vi "Protocol properties.vi"(11 "error in (no error)":errorcluster) -> (8 "LEIN system infor":T1={"STAT system size"=[6, 4, 2, 0, 0, 0, 0, 0, 0, 0, 0, 0, 0, 0, 18, 10]}, 15 "error out":errorcluster)   [LabVIEW 2010]
uses:
  Protocol properties.ctl
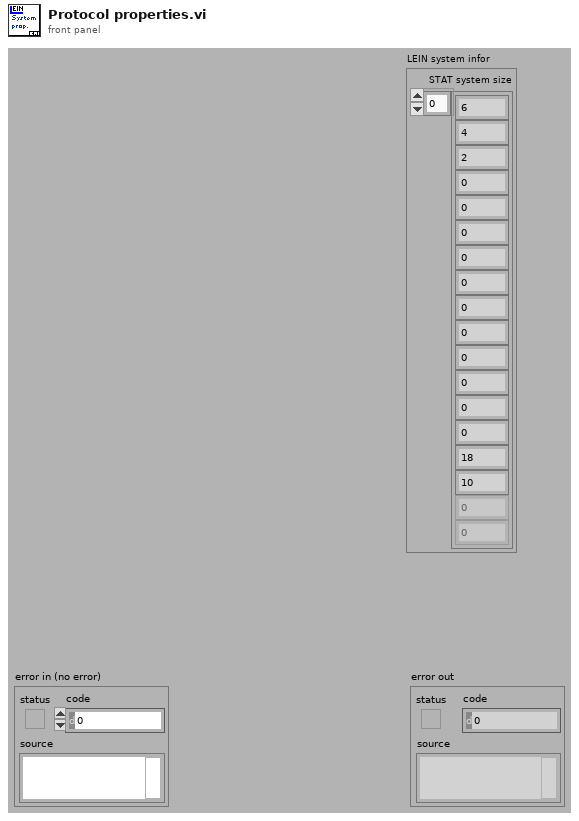
[diagram p1: front panel]
types:
  T1 = typedef "Protocol properties.ctl" = cluster{"STAT system size":u16[]}
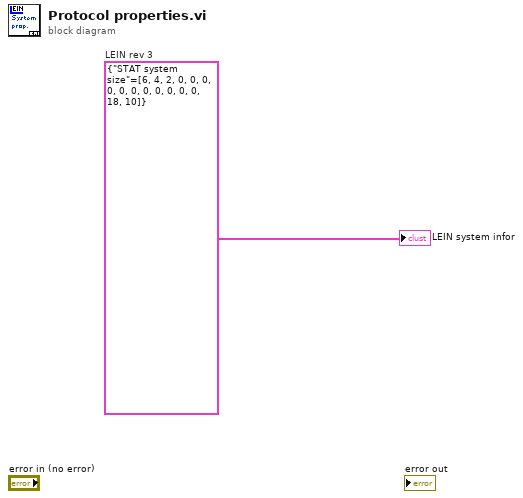
[diagram p0: block diagram]
diagram:
  w1 = T1 {"STAT system size"=[6, 4, 2, 0, 0, 0, 0, 0, 0, 0, 0, 0, 0, 0, 18, 10]}  # LEIN rev 3
  "LEIN system infor" <- w1
